vi "Helium Meter Daemon.vi"() -> ()   [LabVIEW 2015]
uses:
  Libraries/HeliumMonitor/Sensor configuration.ctl
  Libraries/HeliumMonitor/Channel type.ctl
  <vilib>/Platform/TimedLoop/XDataNode/timing_clust.ctl
  <vilib>/Platform/TimedLoop/XDataNode/nitl_modes.ctl
  <vilib>/Platform/TimedLoop/XDataNode/wakeup.ctl
  <vilib>/platform/TimedLoop/XDataNode/XDataNode.xnode
  <vilib>/Platform/TimedLoop/XDataNode/XDNodeRunTimeDep.lvlib
panel:
  out "Dewar level":i32(slide) scale=0.0..1000.0
  in  "Data Folder":path=path "\\\\eden\\NHMFLDATA/Data/nhmflmonitor/Helium/data"
  in  "Tab Control":T1(tab)
  out "History Graph":T2(graph)
  in  "Sensors":T3[](array[typedef])=[{"Name"="Ghz lab", "URL"="http:\\\\130.55.69.25", "Channels"=[{"type"=enum."Flow meter", "number"=6.0}]}, {"Name"="main bag", "URL"="http:\\\\130.55.69.22", "Channels"=[{"type"=enum."Flow meter", "number"=6.0}, {"type"=enum."Tank pressure", "number"=0.0}, {"type"=enum."Dewar level", "number"=1.0}]}, {"Name"="PPMS 20T", "URL"="http:\\\\130.55.69.42", "Channels"=[{"type"=enum."Flow meter", "number"=6.0}]}]
  out "Communication Status":string[](array[string])
  in  "Ignore errors":bool
  out "Helium tank pressure":dbl(knob) scale=0.0..2000.0
  in  "period (ms)":i32=5000
  in  "Display Graph":bool=TRUE
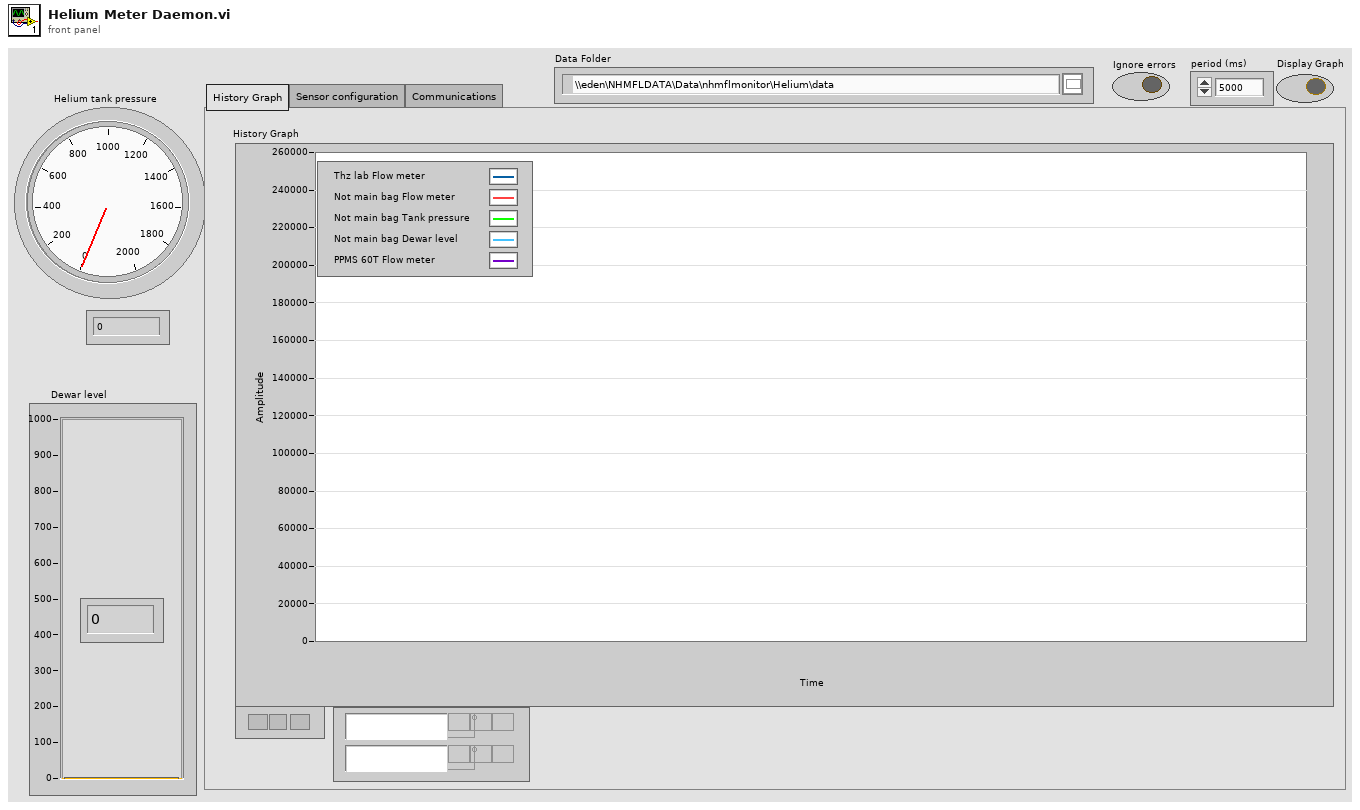
[diagram p1: front panel]
types:
  T1 = enum32{"History Graph", "Sensor configuration", "Communications"}
  T2 = cluster{"output array":dbl[], "output array":dbl[]}[]
  T3 = typedef "Sensor configuration.ctl" = cluster{"Name":string, "URL":string, "Channels":cluster{"type":T4, "number":dbl}[]}
  T4 = typedef "Channel type.ctl" = enum16{"Volts", "Flow meter", "Tank pressure", "Dewar level", "Raw ADC"}
  T5 = typedef "XDNodeRunTimeDep.lvlib/timing_clust.ctl" = cluster{"Expected End [f-1]":u64, "Actual End [f-1]":u64, "Finished Late? [f-1]":bool, "Expected End [i-1]":u64, "Actual End [i-1]":u64, "Finished Late? [i-1]":bool, "Expected Start [i]":u64, "Actual Start [i]":u64, "Expected Start [f]":u64, "Actual Start [f]":u64, "Source Name":string, "Structure Name":string, "Period":i64, "Deadline":i64, "Offset":i64, "Start":i64, "Priority":i32, "Timeout":i32, "Mode":T6, "Wakeup Reason":T7, "Error":errorcluster, "Source Type":string, "Secondary Source Type":string, "Global End Time":u64, "Global Start Time":u64, "Frame Duration":u64, "Iteration Duration":u64, "Assigned CPU":i32, "I/O Scan Engine Mode":u32}
  T6 = typedef "XDNodeRunTimeDep.lvlib/nitl_modes.ctl" = enum32{"No Change", "Process missed periods, maintain original phase", "Discard missed periods, maintain original phase", "Process missed periods, ignore original phase", "Discard missed periods, ignore original phase"}
  T7 = typedef "XDNodeRunTimeDep.lvlib/wakeup.ctl" = enum32{"Normal", "Aborted", "Asynchronous wakeup", "Timing source error", "Timed loop error", "Timeout"}
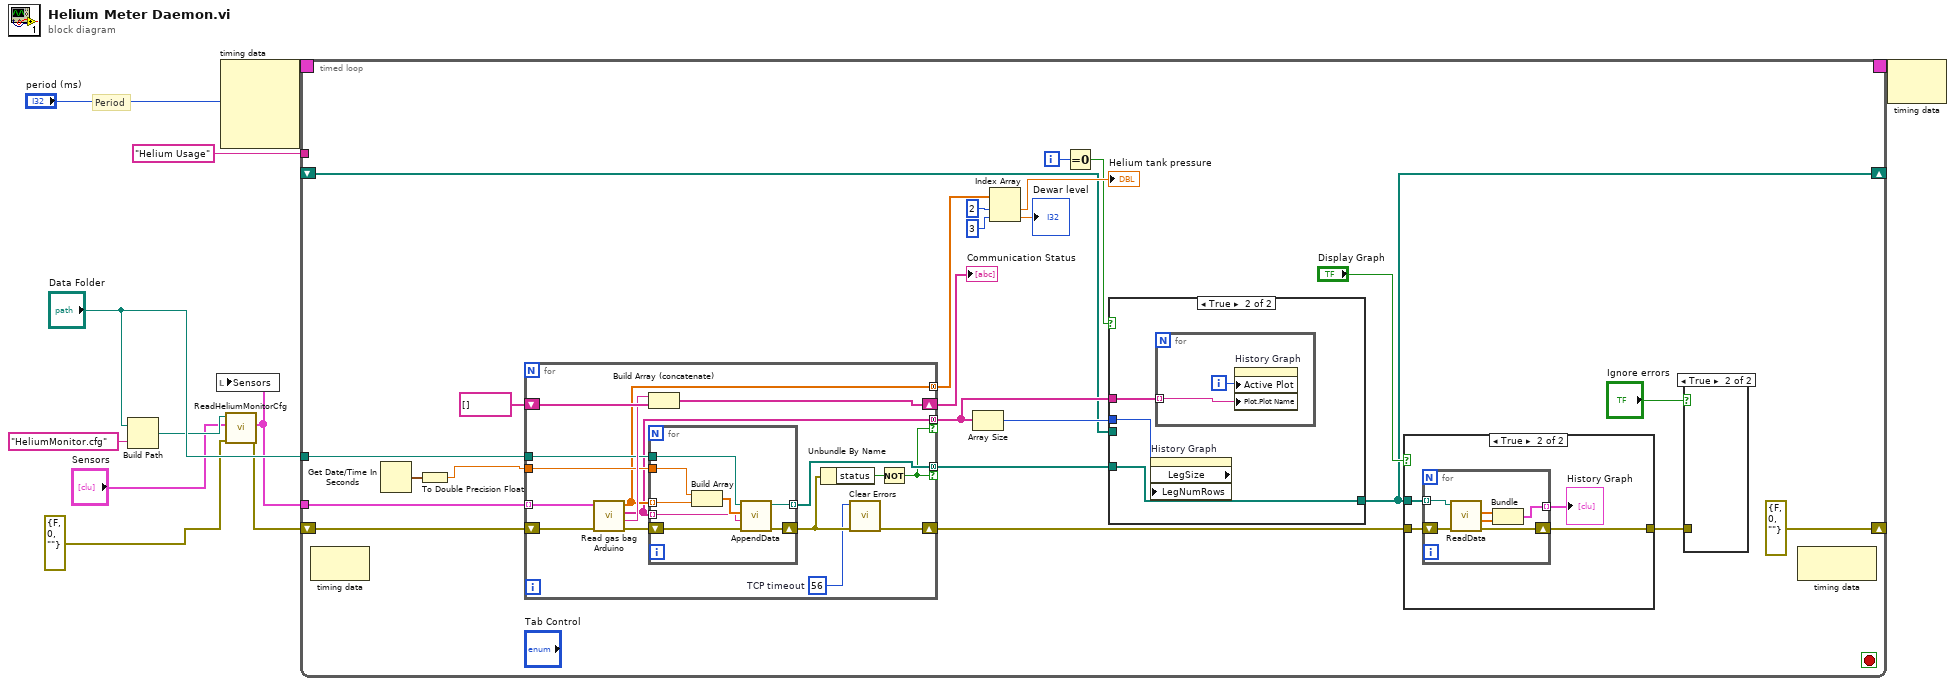
[diagram p0: block diagram]
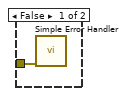
[diagram p3: hidden frame]
diagram:
  # "Period"
  n1 = Build Path(base path="Data Folder", name or relative path="HeliumMonitor.cfg") -> (appended path=w5:path)
  n2 = node-c288("period (ms)") -> (w11:T5)  [unwired: 3 in]
  n3 = call "ReadHeliumMonitorCfg.vi"("Error In"=errorcluster {"status"=FALSE, "code"=0, "source"=""} ("error out"), "Sensors"="Sensors", "CFG File Path"=w5) -> ("Error Out"=w2:errorcluster, "Sensors out"=w1:T3[])  [unwired: 6 in, 1 out]
  n4 = local write "Sensors"(w1) -> ()
  n5 = timed-loop {
    timing: w11 -> [_]
    timing-out: [_] -> w10
    tunnel: "Data Folder" -> [w21]
    tunnel: "Helium Usage" -> [_]
    shift-right: [errorcluster {"status"=FALSE, "code"=0, "source"=""} ("error out")] -> _
    shift-left: w2 -> [w33]
    shift-right: [w13] -> _
    shift-left: _ -> [w14]
    tunnel: w1 -> [w12]
    i -> [w26]
    stop <- _ stop-if-true
    n6 = node-c288() -> ()  [unwired: 1 in, 1 out]
    n7 = Get Date/Time In Seconds() -> (seconds since 1Jan1904=w34:timestamp)
    n8 = To Double Precision Float(number=w34) -> (double precision float=w20:dbl)
    n9 = for {
      tunnel: w12 -> [w57] mode=indexing
      shift-right: [w44] -> w19
      shift-left: w33 -> [w58]
      tunnel: [w51] -> w24 mode=concatenating
      tunnel: [w50] -> w17 mode=concatenating if=w46
      shift-right: [w56] -> w22
      shift-left: string[] [] -> [w55]
      tunnel: w21 -> [w53]
      tunnel: w20 -> [w52]
      tunnel: [w47] -> w15 mode=concatenating if=w46
      w43 = 56  # TCP timeout
      n10 = call "Read gas bag Arduino.vi"("Sensor configuration"=w57, "Error In"=w58) -> ("Data"=w51:dbl[], "Names"=w50:string[], "Communication error"=w54:string, "Error Out"=w49:errorcluster)  [unwired: 5 in]
      n11 = Build Array (concatenate)(w54, w55) -> (w56:string[])
      n12 = for {
        shift-right: [w65] -> w45
        shift-left: w49 -> [w64]
        tunnel: w52 -> [w63]
        tunnel: w53 -> [w66]
        tunnel: [w61] -> w47 mode=indexing
        tunnel: w51 -> [w60] mode=indexing
        tunnel: w50 -> [w59] mode=indexing
        n13 = Build Array(w63, w60) -> (w62:dbl[])
        n14 = call "AppendData.vi"("Error In"=w64, "Name"=w59, "Data"=w62, "Folder"=w66) -> ("Error Out"=w65:errorcluster, "File Path Control out"=w61:path)  [unwired: 6 in]
      }
      n15 = Unbundle By Name(w45) -> ("status"=w48:bool)
      n16 = call <vilib>:"Clear Errors.vi"("error in (no error)"=w45, "specific error code to clear (0: all)"=w43) -> ("error out"=w44:errorcluster)  [unwired: 4 in, 1 out]
      n17 = Not(x=w48) -> (.not. x?=w46:bool)
    }
    "Communication Status" <- w22
    n18 = Array Size(array=w17) -> (size(s)=w18:i32)
    n19 = Index Array(array=w24, index #1=2 ("index"), index #2=3 ("index")) -> (element #1=→"Helium tank pressure":dbl, element #2=→"Dewar level":dbl)
    n20 = Equal To 0?(x=w26) -> (x = 0?=w16:bool)
    n21 = case shown="True" w16 {
      tunnel: w17 -> [_ w39]
      tunnel: w18 -> [_ w38]
      tunnel: w15 -> [_ w37]
      tunnel: [w36 w37] -> w13
      tunnel: w14 -> [w36 _]
      frame False {
      }
      frame True {
        n22 = property on="History Graph" class="XYGraph (strict)" props=["LegSize", "LegNumRows"]("LegNumRows"=w38) -> ()  [unwired: 2 in, 3 out]
        n23 = for {
          tunnel: w39 -> [w41] mode=indexing
          i -> [w40]
          n24 = property on="History Graph" class="XYGraph (strict)"("Active Plot"=w40, "Plot.Plot Name"=w41) -> ()  [unwired: 2 in, 2 out]
        }
      }
    }
    n25 = case shown="True" "Display Graph" {
      tunnel: w13 -> [_ w68]
      tunnel: w19 -> [w67 w71]
      tunnel: [w67 w70] -> w31
      frame False {
      }
      frame True {
        n26 = for {
          shift-right: [w76] -> w70
          shift-left: w71 -> [w77]
          tunnel: [w75] -> w69 mode=indexing
          tunnel: w68 -> [w72] mode=indexing
          n27 = call "ReadData.vi"("Error In"=w77, "File Path Control"=w72) -> ("Error Out"=w76:errorcluster, "Y"=w73:dbl[], "X"=w74:dbl[])  [unwired: 6 in, 1 out]
          n28 = Bundle("X"=w74, "Y"=w73) -> (w75:cluster{"X":dbl[], "Y":dbl[]})  [unwired: 1 in]
        }
        "History Graph" <- w69
      }
    }
    n29 = case shown="True" "Ignore errors" {
      tunnel: w31 -> [w42 _]
      frame False {
        n30 = call <vilib>:"Simple Error Handler.vi"("error in (no error)"=w42) -> ()  [unwired: 4 in, 5 out]
      }
      frame True {
      }
    }
    n31 = node-c288() -> ()  [unwired: 1 in, 1 out]
  }
  n32 = node-c288(w10) -> ()  [unwired: 1 out]
